vi "Read N Key Tap Positions.vi"(8 "Error In":errorcluster, 11 "Leap Handle":T2) -> (0 "Error Out":errorcluster, 1 "Key Tap Statuses":T1[](array[typedef]), 2 "Key Tap Positions":cluster{"X":sgl, "Y":sgl, "Z":sgl}[](array[cluster]), 3 "Leap Handle":T2)   [LabVIEW 2011, in "LVH-Leap.lvlib"]
doc: "Read N key tap gesture positions."
uses:
  LVH-Leap.lvlib
  Private/Type Defs/Leap Handle.ctl
  C:/github/labviewhacker/LVH-Leap/LabVIEW/vi.lib/LabVIEW Hacker/Leap/Private/Libs/LeapCSharp.NET3.5.dll
  Private/Libs/LeapCSharp.NET3.5.dll
  Private/Type Defs/Gesture State.ctl
  Read N Key Taps.vi
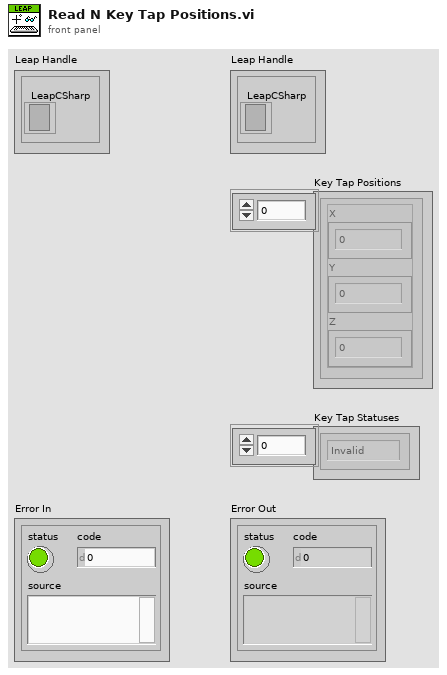
[diagram p1: front panel]
types:
  T1 = typedef "LVH-Leap.lvlib/Gesture State.ctl" = enum16{"Invalid", "Start", "Update", "Stop"}
  T2 = typedef "LVH-Leap.lvlib/Leap Handle.ctl" = cluster{"LeapCSharp":refnum<k24>}
  T3 = typedef "LVH-Leap.lvlib/Gesture Key Tap.ctl" = cluster{"Common":T4, "Direction":T6, "Position":T6, "Progress":dbl}
  T4 = typedef "LVH-Leap.lvlib/Gesture Common.ctl" = cluster{"ID":dbl, "Duration (S)":dbl, "Gesture Type":T5, "Gesture State":T1}
  T5 = typedef "LVH-Leap.lvlib/Gesture Type.ctl" = enum16{"Invalid", "Swipe", "Circle", "Screen Tap", "Key Tap"}
  T6 = typedef "LVH-Leap.lvlib/Vector.ctl" = cluster{"Pitch":sgl, "Yaw":sgl, "Roll":sgl, "Magnitude":sgl, "XYZ":sgl[]}
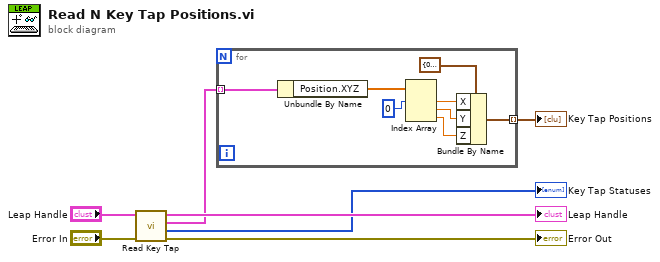
[diagram p0: block diagram]
diagram:
  n1 = call-poly "Read Key Tap.vi"("Error In"="Error In", "Leap Handle"="Leap Handle") -> ("Error Out"=→"Error Out":errorcluster, "Key Tap Statuses"=→"Key Tap Statuses":T1[], "Key Tap Gestures"=w2:T3[], "Leap Handle"=→"Leap Handle":T2)  [unwired: 6 in]
  n2 = for {
    tunnel: w2 -> [w15] mode=indexing
    tunnel: [w8] -> w1 mode=indexing
    n3 = Unbundle By Name(w15) -> ("Position.XYZ"=w14:sgl[])
    n4 = Index Array(array=w14, index #1=0 ("index")) -> (element #1=w11:sgl, element #2=w10:sgl, element #3=w9:sgl)  [unwired: 2 in]
    n5 = Bundle By Name(cluster=cluster{"X":sgl, "Y":sgl, "Z":sgl} {"X"=0.0, "Y"=0.0, "Z"=0.0}, "X"=w11, "Y"=w10, "Z"=w9) -> (w8:cluster{"X":sgl, "Y":sgl, "Z":sgl})
  }
  "Key Tap Positions" <- w1
